vi "Set Intensity Graph Y Scale Array.vi"(8 "error in (no error)":errorcluster, 10 "Y Scale":dbl[](array[numeric]), 11 "graph_utilities in":refnum<class "graph_utilities.lvclass">) -> (0 "error out":errorcluster, 3 "graph_utilities out":refnum<class "graph_utilities.lvclass">)   [LabVIEW 2016, in "graph_utilities.lvclass"]
doc: "Set the Y Offset and Multiple of the Intensity Graph by wiring an array to Y Scale"
uses:
  graph_utilities.lvclass
  graph_utilities.lvclass/graph_utilities.ctl
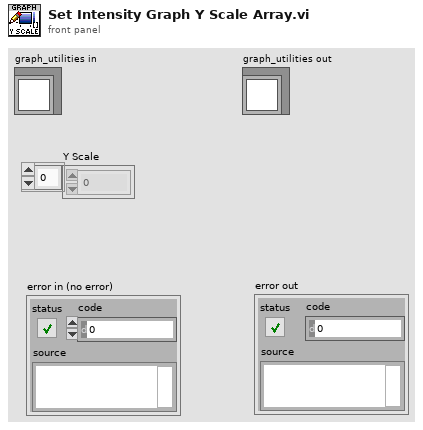
[diagram p1: front panel]
types:
  T1 = typedef "LVOffsetAndMultiplierTypeDef.ctl" = cluster{"Offset":dbl, "Multiplier":dbl}
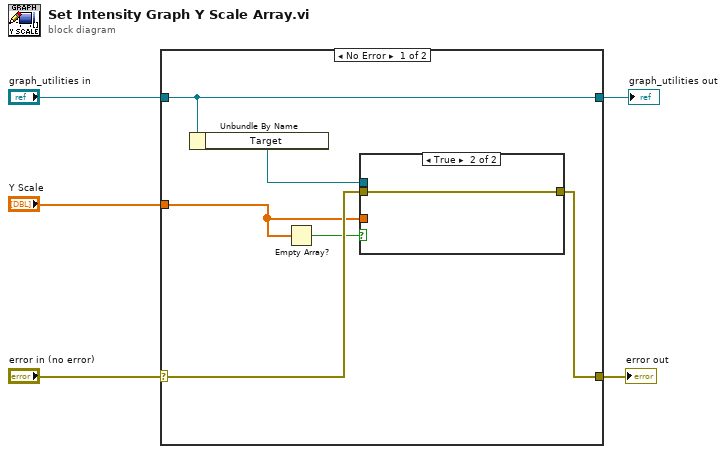
[diagram p0: block diagram]
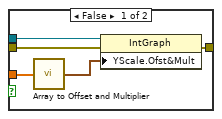
[diagram p2: hidden frame]
diagram:
  n1 = case shown="No Error" "error in (no error)" {
    selector: "error in (no error)" -> [w10 w19]
    tunnel: "Y Scale" -> [w8 _]
    tunnel: [w11 w19] -> w4
    tunnel: "graph_utilities in" -> [w9 w18]
    tunnel: [w9 w18] -> w1
    frame No Error {
      n2 = Unbundle By Name(w9) -> ("Target"=w7:refnum<vi>)
      n3 = Empty Array?(array=w8) -> (empty?=w6:bool)
      n4 = case shown="True" w6 {
        tunnel: [w16 w17] -> w11
        tunnel: w10 -> [w15 w17]
        tunnel: w8 -> [w14 _]
        tunnel: w7 -> [w12 _]
        frame False {
          n5 = call "Array to Offset and Multiplier.vi"("Array"=w14) -> ("Offset and Multiplier"=w13:T1)
          n6 = property on="Property Node" class="IntGraph"(reference=w12, error in=w15, "YScale.Ofst&Mult"=w13) -> (error out=w16:errorcluster)  [unwired: 1 out]
        }
        frame True {
        }
      }
    }
    frame Error {
    }
  }
  "error out" <- w4
  "graph_utilities out" <- w1
